vi "Build DashBoard Data.vi"(11 "Dashboard Enables":T3={"Analog Module 1"=[TRUE, TRUE, TRUE, TRUE, TRUE, TRUE, TRUE, TRUE], "Analog Module 2"=[FALSE, FALSE, FALSE, FALSE, FALSE, FALSE, FALSE, FALSE], "Digital Module 1"=TRUE, "Digital Module 2"=FALSE, "Solenoid Module"=TRUE}) -> ()   [LabVIEW 2011]
doc: "This VI builds data and sends it back to the dashboard PC program. By default it sends back the raw values for the first analog, digital, and solenoid module. Modify it to send back the data you want to view. Consider adding higher level data to the Dashboard Datatype.ctl and to this VI. Then update the Dashboard to display the data however you like.\n\nThis software is licensed. Open the labview\\readme\\WPI Robotics Library Open Source License.txt file for more information."
uses:
  DashboardEnable.ctl
  Dashboard Datatype.ctl
  <vilib>/Rock Robotics/WPI/DriverStation/WPI_DriverStationDigitalData.ctl
  <vilib>/Rock Robotics/WPI/DriverStation/DriverStationLCD/WPI_DriverStationLCDLCDLine.ctl
  System Set Points and States.vi
  Robot Global Data.vi
panel:
  out "Dashboard Data":T1
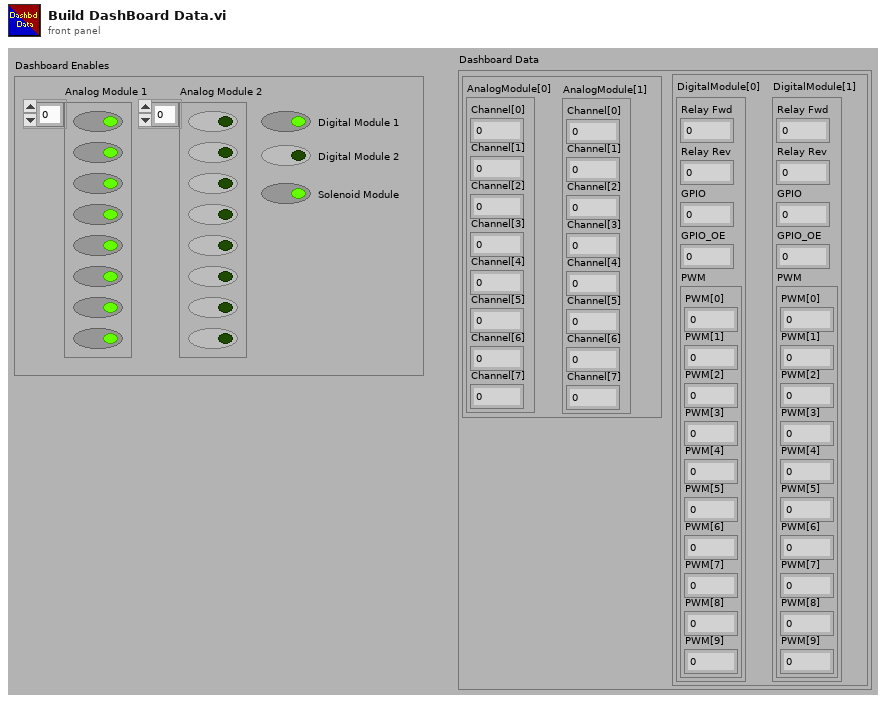
[diagram p1: front panel]
types:
  T1 = typedef "Dashboard Datatype.ctl" = cluster{cluster{"AnalogModule[0]":cluster{"Channel[0]":sgl, "Channel[1]":sgl, "Channel[2]":sgl, "Channel[3]":sgl, "Channel[4]":sgl, "Channel[5]":sgl, "Channel[6]":sgl, "Channel[7]":sgl}, "AnalogModule[1]":cluster{"Channel[0]":sgl, "Channel[1]":sgl, "Channel[2]":sgl, "Channel[3]":sgl, "Channel[4]":sgl, "Channel[5]":sgl, "Channel[6]":sgl, "Channel[7]":sgl}}, cluster{"DigitalModule[0]":T2, "DigitalModule[1]":T2}}
  T2 = typedef "WPI_DriverStationDigitalData.ctl" = cluster{"Relay Fwd":u8, "Relay Rev":u8, "GPIO":u16, "GPIO_OE":u16, "PWM":cluster{"PWM[0]":u8, "PWM[1]":u8, "PWM[2]":u8, "PWM[3]":u8, "PWM[4]":u8, "PWM[5]":u8, "PWM[6]":u8, "PWM[7]":u8, "PWM[8]":u8, "PWM[9]":u8}}
  T3 = typedef "DashboardEnable.ctl" = cluster{"Analog Module 1":bool[], "Analog Module 2":bool[], "Digital Module 1":bool, "Digital Module 2":bool, "Solenoid Module":bool}
  T4 = typedef "WPI_DriverStationLCDLCDLine.ctl" = enum16{"Main - Line 1", "User - Line 2", "User - Line 3", "User - Line 4", "User - Line 5", "User - Line 6"}
  T5 = cluster{"Position":cluster{"X":dbl, "Y":dbl}, "Distance (ft)":dbl}[]
  T6 = cluster{"Target Info[0]":cluster{"Position":cluster{"X":dbl, "Y":dbl}, "Distance (ft)":dbl}, "Target Info[1]":cluster{"Position":cluster{"X":dbl, "Y":dbl}, "Distance (ft)":dbl}, "Target Info[2]":cluster{"Position":cluster{"X":dbl, "Y":dbl}, "Distance (ft)":dbl}, "Target Info[3]":cluster{"Position":cluster{"X":dbl, "Y":dbl}, "Distance (ft)":dbl}, "Target Info[4]":cluster{"Position":cluster{"X":dbl, "Y":dbl}, "Distance (ft)":dbl}, "Target Info[5]":cluster{"Position":cluster{"X":dbl, "Y":dbl}, "Distance (ft)":dbl}, "Target Info[6]":cluster{"Position":cluster{"X":dbl, "Y":dbl}, "Distance (ft)":dbl}, "Target Info[7]":cluster{"Position":cluster{"X":dbl, "Y":dbl}, "Distance (ft)":dbl}, "Target Info[8]":cluster{"Position":cluster{"X":dbl, "Y":dbl}, "Distance (ft)":dbl}}
  T7 = cluster{"AnalogModule[0]":cluster{"Channel[0]":sgl, "Channel[1]":sgl, "Channel[2]":sgl, "Channel[3]":sgl, "Channel[4]":sgl, "Channel[5]":sgl, "Channel[6]":sgl, "Channel[7]":sgl}, "AnalogModule[1]":cluster{"Channel[0]":sgl, "Channel[1]":sgl, "Channel[2]":sgl, "Channel[3]":sgl, "Channel[4]":sgl, "Channel[5]":sgl, "Channel[6]":sgl, "Channel[7]":sgl}}
  T8 = cluster{"Channel[0]":sgl, "Channel[1]":sgl, "Channel[2]":sgl, "Channel[3]":sgl, "Channel[4]":sgl, "Channel[5]":sgl, "Channel[6]":sgl, "Channel[7]":sgl}[]
  T9 = cluster{"Channel[0]":sgl, "Channel[1]":sgl, "Channel[2]":sgl, "Channel[3]":sgl, "Channel[4]":sgl, "Channel[5]":sgl, "Channel[6]":sgl, "Channel[7]":sgl}
  T10 = cluster{"AnalogModule[0][0]":sgl, "AnalogModule[0][1]":sgl, "AnalogModule[0][2]":sgl, "AnalogModule[0][3]":sgl, "AnalogModule[0][4]":sgl, "AnalogModule[0][5]":sgl, "AnalogModule[0][6]":sgl, "AnalogModule[0][7]":sgl}
  T11 = cluster{"[0]":cluster{"Channel[0]":sgl, "Channel[1]":sgl, "Channel[2]":sgl, "Channel[3]":sgl, "Channel[4]":sgl, "Channel[5]":sgl, "Channel[6]":sgl, "Channel[7]":sgl}, "[1]":cluster{"Channel[0]":sgl, "Channel[1]":sgl, "Channel[2]":sgl, "Channel[3]":sgl, "Channel[4]":sgl, "Channel[5]":sgl, "Channel[6]":sgl, "Channel[7]":sgl}}
  T12 = cluster{"DigitalModule[0]":T2, "DigitalModule[1]":T2}
  T13 = typedef "FPGA_DIODevRef.ctl" = cluster{"DevStatus":errorcluster, "Module":T14}
  T14 = typedef "FPGA_TypedefDigitalModule.ctl" = enum16{"Digital Module 1", "Digital Module 2"}
  T15 = cluster{"[0]":u8, "[1]":u8, "[2]":u8, "[3]":u8, "[4]":u8, "[5]":u8, "[6]":u8, "[7]":u8, "[8]":u8, "[9]":u8}
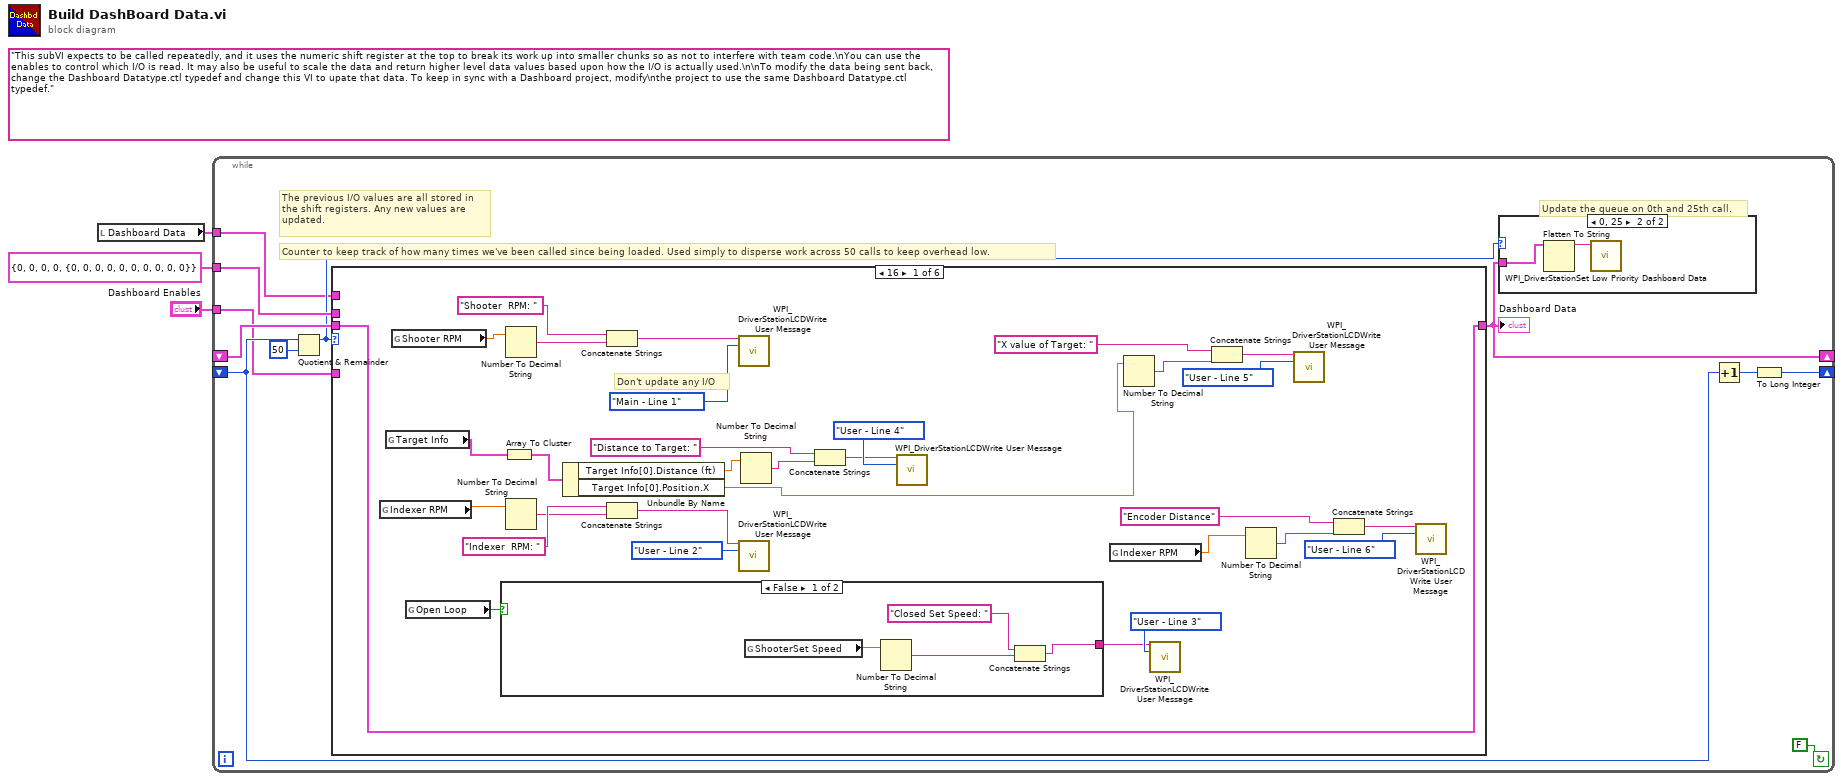
[diagram p0: block diagram]
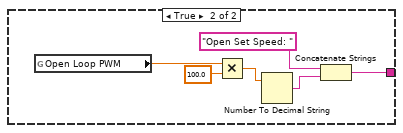
[diagram p3: hidden frame]
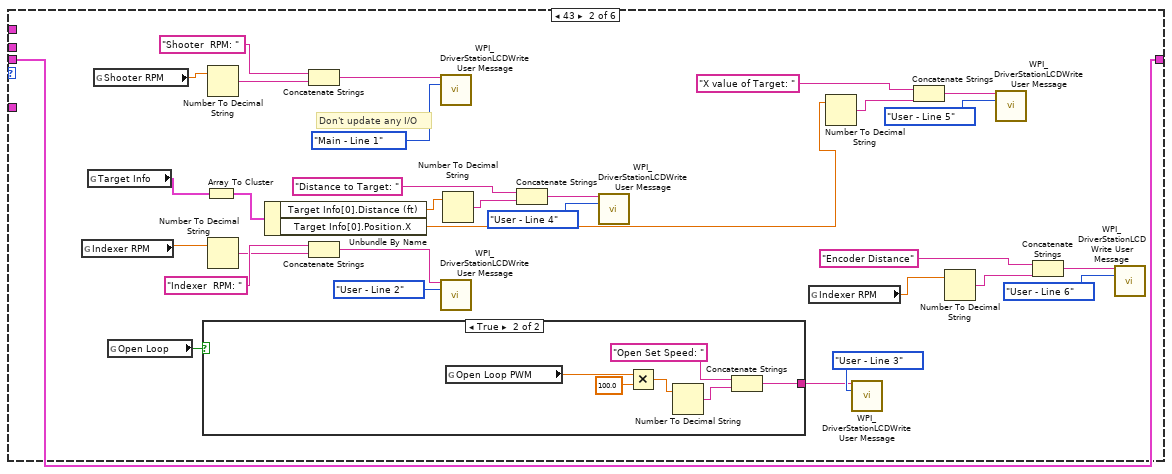
[diagram p4: hidden frame]
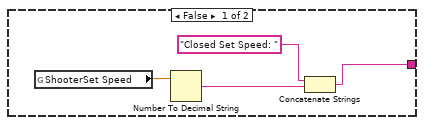
[diagram p5: hidden frame]
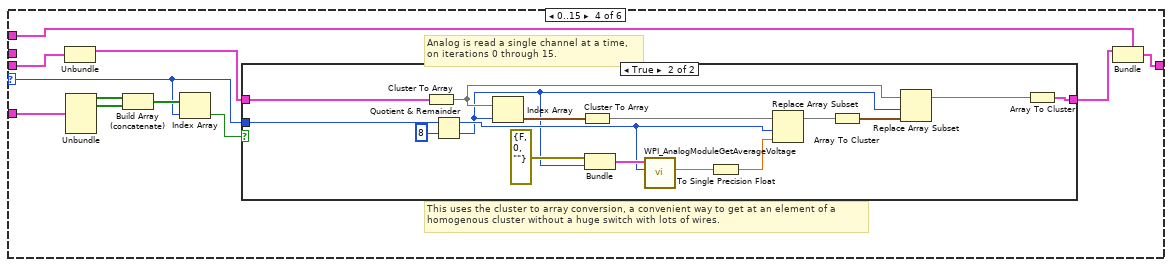
[diagram p7: hidden frame]
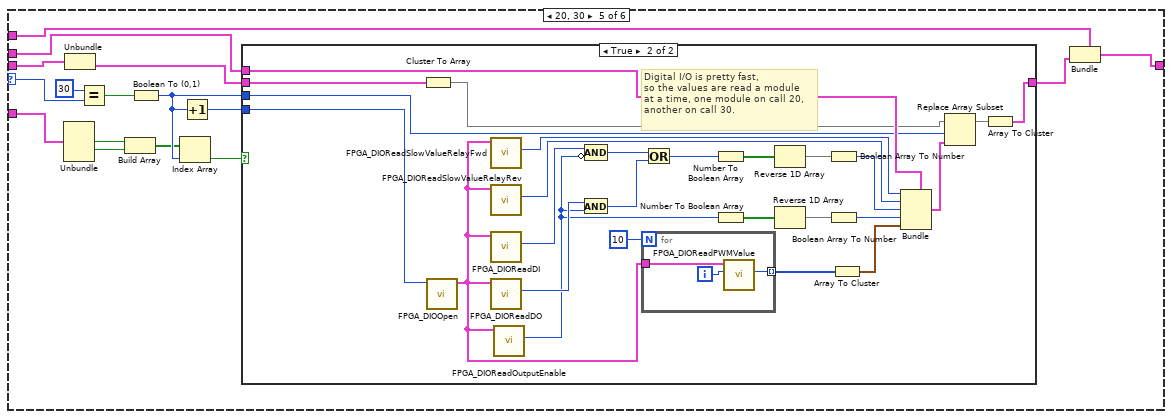
[diagram p9: hidden frame]
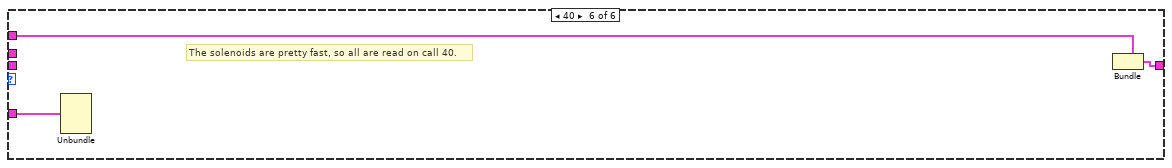
[diagram p11: hidden frame]
diagram:
  (unwired) "This subVI expects to be called repeatedly, and it uses the numeric shift register at the top to break its work up into smaller chunks so as not to interfere with team code.\nYou can use the enables to control which I/O is read. It may also be useful to scale the data and return higher level data values based upon how the I/O is actually used.\n\nTo modify the data being sent back, change the Dashboard Datatype.ctl typedef and change this VI to upate that data. To keep in sync with a Dashboard project, modify\nthe project to use the same Dashboard Datatype.ctl typedef."
  n1 = local read "Dashboard Data"() -> (w2:T1)
  n2 = while {
    shift-right: [w7] -> _
    shift-left: _ -> [w9]
    shift-right: [w4] -> _
    shift-left: _ -> [w12]
    tunnel: T2 {"Relay Fwd"=0, "Relay Rev"=0, "GPIO"=0, "GPIO_OE"=0, "PWM"={"PWM[0]"=0, "PWM[1]"=0, "PWM[2]"=0, "PWM[3]"=0, "PWM[4]"=0, "PWM[5]"=0, "PWM[6]"=0, "PWM[7]"=0, "PWM[8]"=0, "PWM[9]"=0}} ("DigitalModule[1]") -> [w11]
    tunnel: w2 -> [w6]
    tunnel: "Dashboard Enables" -> [w5]
    stop <- FALSE continue-if-true
    # "Counter to keep track of how many times we've been called since being loaded. Used simply to disperse work across 50 calls to keep overhead low."
    # "Update the queue on 0th and 25th call."
    # "The previous I/O values are all stored in\nthe shift registers. Any new values are\nupdated."
    n3 = Quotient & Remainder(x=w9, y=50) -> (x-y*floor(x/y)=w8:i32)  [unwired: 1 out]
    n4 = case shown="16" w8 {
      selector: w8 -> [_ _ _ w105 w137 _]
      tunnel: [w47 w63 w99 w101 w128 w175] -> w4
      tunnel: w12 -> [w47 w63 w99 w100 w130 _]
      tunnel: w11 -> [_ _ _ _ w143 _]
      tunnel: w6 -> [_ _ _ w107 w129 w174]
      tunnel: w5 -> [_ _ _ w104 w135 w176]
      frame 16 {
        # "Don't update any I/O"
        n5 = global read "System Set Points and States.vi" "Indexer RPM"() -> (w31:dbl)
        n6 = global read "Robot Global Data.vi" "Target Info"() -> (w39:T5)
        n7 = global read "System Set Points and States.vi" "Shooter RPM"() -> (w30:dbl)
        n8 = global read "System Set Points and States.vi" "Open Loop"() -> (w46:bool)
        n9 = case shown="False" w46 {
          tunnel: [w50 w57] -> w44
          frame False {
            n10 = global read "System Set Points and States.vi" "ShooterSet Speed"() -> (w48:dbl)
            n11 = Number To Decimal String(number=w48) -> (decimal integer string=w49:string)  [unwired: 1 in]
            n12 = Concatenate Strings("Closed Set Speed: ", w49) -> (w50:string)
          }
          frame True {
            n13 = global read "System Set Points and States.vi" "Open Loop PWM"() -> (w56:dbl)
            n14 = Multiply(x=w56, y=100.0) -> (x*y=w52:dbl)
            n15 = Number To Decimal String(number=w52) -> (decimal integer string=w53:string)  [unwired: 1 in]
            n16 = Concatenate Strings("Open Set Speed: " ("string"), w53) -> (w57:string)
          }
        }
        n17 = Array To Cluster(array=w39) -> (cluster=w26:T6)
        n18 = Number To Decimal String(number=w30) -> (decimal integer string=w40:string)  [unwired: 1 in]
        n19 = Number To Decimal String(number=w31) -> (decimal integer string=w32:string)  [unwired: 1 in]
        n20 = Unbundle By Name(w26) -> ("Target Info[0].Distance (ft)"=w23:dbl, "Target Info[0].Position.X"=w25:dbl)
        n21 = Concatenate Strings("Shooter  RPM: ", w40) -> (w42:string)
        n22 = Concatenate Strings("Indexer  RPM: ", w32) -> (w34:string)
        n23 = call <vilib>:"WPI_DriverStationLCDWrite User Message.vi"("line text"=w42, "line"=WPI_DriverStationLCDLCDLine."Main - Line 1") -> ()  [unwired: 13 in, 1 out]
        n24 = call <vilib>:"WPI_DriverStationLCDWrite User Message.vi"("line text"=w34, "line"=WPI_DriverStationLCDLCDLine."User - Line 2") -> ()  [unwired: 13 in, 1 out]
        n25 = Number To Decimal String(number=w23) -> (decimal integer string=w22:string)  [unwired: 1 in]
        n26 = Concatenate Strings("Distance to Target: " ("string"), w22) -> (w36:string)
        n27 = call <vilib>:"WPI_DriverStationLCDWrite User Message.vi"("line text"=w36, "line"=WPI_DriverStationLCDLCDLine."User - Line 4") -> ()  [unwired: 13 in, 1 out]
        n28 = global read "System Set Points and States.vi" "Indexer RPM"() -> (w17:dbl)
        n29 = Number To Decimal String(number=w25) -> (decimal integer string=w24:string)  [unwired: 1 in]
        n30 = call <vilib>:"WPI_DriverStationLCDWrite User Message.vi"("line text"=w44, "line"=WPI_DriverStationLCDLCDLine."User - Line 3") -> ()  [unwired: 13 in, 1 out]
        n31 = Concatenate Strings("X value of Target: " ("string"), w24) -> (w27:string)
        n32 = Number To Decimal String(number=w17) -> (decimal integer string=w18:string)  [unwired: 1 in]
        n33 = call <vilib>:"WPI_DriverStationLCDWrite User Message.vi"("line text"=w27, "line"=WPI_DriverStationLCDLCDLine."User - Line 5") -> ()  [unwired: 13 in, 1 out]
        n34 = Concatenate Strings("Encoder Distance" ("string"), w18) -> (w19:string)
        n35 = call <vilib>:"WPI_DriverStationLCDWrite User Message.vi"("line text"=w19, "line"=WPI_DriverStationLCDLCDLine."User - Line 6") -> ()  [unwired: 13 in, 1 out]
      }
      frame 43 {
        # "Don't update any I/O"
        n36 = global read "System Set Points and States.vi" "Indexer RPM"() -> (w73:dbl)
        n37 = global read "Robot Global Data.vi" "Target Info"() -> (w81:T5)
        n38 = global read "System Set Points and States.vi" "Shooter RPM"() -> (w72:dbl)
        n39 = global read "System Set Points and States.vi" "Open Loop"() -> (w88:bool)
        n40 = case shown="True" w88 {
          tunnel: [w89 w98] -> w86
          frame False {
            n41 = global read "System Set Points and States.vi" "ShooterSet Speed"() -> (w90:dbl)
            n42 = Number To Decimal String(number=w90) -> (decimal integer string=w91:string)  [unwired: 1 in]
            n43 = Concatenate Strings("Closed Set Speed: ", w91) -> (w89:string)
          }
          frame True {
            n44 = global read "System Set Points and States.vi" "Open Loop PWM"() -> (w97:dbl)
            n45 = Multiply(x=w97, y=100.0) -> (x*y=w93:dbl)
            n46 = Number To Decimal String(number=w93) -> (decimal integer string=w94:string)  [unwired: 1 in]
            n47 = Concatenate Strings("Open Set Speed: " ("string"), w94) -> (w98:string)
          }
        }
        n48 = Array To Cluster(array=w81) -> (cluster=w68:T6)
        n49 = Number To Decimal String(number=w72) -> (decimal integer string=w82:string)  [unwired: 1 in]
        n50 = Number To Decimal String(number=w73) -> (decimal integer string=w74:string)  [unwired: 1 in]
        n51 = Unbundle By Name(w68) -> ("Target Info[0].Distance (ft)"=w65:dbl, "Target Info[0].Position.X"=w67:dbl)
        n52 = Concatenate Strings("Shooter  RPM: ", w82) -> (w84:string)
        n53 = Concatenate Strings("Indexer  RPM: ", w74) -> (w76:string)
        n54 = call <vilib>:"WPI_DriverStationLCDWrite User Message.vi"("line text"=w84, "line"=WPI_DriverStationLCDLCDLine."Main - Line 1") -> ()  [unwired: 13 in, 1 out]
        n55 = call <vilib>:"WPI_DriverStationLCDWrite User Message.vi"("line text"=w76, "line"=WPI_DriverStationLCDLCDLine."User - Line 2") -> ()  [unwired: 13 in, 1 out]
        n56 = Number To Decimal String(number=w65) -> (decimal integer string=w64:string)  [unwired: 1 in]
        n57 = Concatenate Strings("Distance to Target: " ("string"), w64) -> (w78:string)
        n58 = call <vilib>:"WPI_DriverStationLCDWrite User Message.vi"("line text"=w78, "line"=WPI_DriverStationLCDLCDLine."User - Line 4") -> ()  [unwired: 13 in, 1 out]
        n59 = global read "System Set Points and States.vi" "Indexer RPM"() -> (w58:dbl)
        n60 = Number To Decimal String(number=w67) -> (decimal integer string=w66:string)  [unwired: 1 in]
        n61 = call <vilib>:"WPI_DriverStationLCDWrite User Message.vi"("line text"=w86, "line"=WPI_DriverStationLCDLCDLine."User - Line 3") -> ()  [unwired: 13 in, 1 out]
        n62 = Concatenate Strings("X value of Target: " ("string"), w66) -> (w69:string)
        n63 = Number To Decimal String(number=w58) -> (decimal integer string=w59:string)  [unwired: 1 in]
        n64 = call <vilib>:"WPI_DriverStationLCDWrite User Message.vi"("line text"=w69, "line"=WPI_DriverStationLCDLCDLine."User - Line 5") -> ()  [unwired: 13 in, 1 out]
        n65 = Concatenate Strings("Encoder Distance" ("string"), w59) -> (w60:string)
        n66 = call <vilib>:"WPI_DriverStationLCDWrite User Message.vi"("line text"=w60, "line"=WPI_DriverStationLCDLCDLine."User - Line 6") -> ()  [unwired: 13 in, 1 out]
      }
      frame Default {
      }
      frame 0..15 {
        # "This uses the cluster to array conversion, a convenient way to get at an element of a\nhomogenous cluster without a huge switch with lots of wires."
        # "Analog is read a single channel at a time,\non iterations 0 through 15."
        n67 = Unbundle(w100) -> (w106:T7)  [unwired: 1 out]
        n68 = Unbundle(w104) -> ("Analog Module 1"=w103:bool[], "Analog Module 2"=w102:bool[])  [unwired: 3 out]
        n69 = Build Array (concatenate)(w103, w102) -> (w109:bool[])
        n70 = Index Array(array=w109, index=w105) -> (element=w110:bool)
        n71 = case shown="True" w110 {
          tunnel: w105 -> [_ w118]
          tunnel: [w111 w115] -> w108
          tunnel: w106 -> [w111 w114]
          frame False {
          }
          frame True {
            n72 = Cluster To Array(cluster=w114) -> (array=w113:T8)
            n73 = Quotient & Remainder(x=w118, y=8) -> (x-y*floor(x/y)=w117:i32, floor(x/y)=w112:i32)
            n74 = Index Array(array=w113, index=w112) -> (element=w120:T9)
            n75 = Cluster To Array(cluster=w120) -> (array=w119:sgl[])
            n76 = Bundle("DevStatus"=errorcluster {"status"=FALSE, "code"=0, "source"=""}, w112) -> (w126:cluster{"DevStatus":errorcluster, i32})  [unwired: 1 out]
            n77 = call <vilib>:"WPI_AnalogModuleGetAverageVoltage.vi"("Channel"=w117, "AnalogModuleDevStatus"=w126) -> ("Average Voltage"=w123:dbl)  [unwired: 1 in, 8 out]
            n78 = To Single Precision Float(number=w123) -> (single precision float=w122:sgl)
            n79 = Replace Array Subset(array=w119, new element=w122, index=w117) -> (w121:sgl[])
            n80 = Array To Cluster(array=w121) -> (cluster=w125:T10)
            n81 = Replace Array Subset(array=w113, new element=w125, index=w112) -> (w116:T8)
            n82 = Array To Cluster(array=w116) -> (cluster=w115:T11)
          }
        }
        n83 = Bundle(cluster=w107, w108) -> (w101:T1)  [unwired: 1 out]
      }
      frame 20, 30 {
        n84 = Unbundle(w135) -> ("Digital Module 1"=w134:bool, "Digital Module 2"=w133:bool)  [unwired: 3 out]
        n85 = Unbundle(w130) -> (w132:T12)  [unwired: 1 out]
        n86 = Equal?(x=30, y=w137) -> (x = y?=w141:bool)
        n87 = Build Array(w134, w133) -> (w136:bool[])
        n88 = Boolean To (0,1)(Boolean=w141) -> (0, 1=w139:i16)
        n89 = Index Array(array=w136, index=w139) -> (element=w138:bool)
        n90 = Increment(x=w139) -> (x+1=w140:i16)
        n91 = case shown="True" w138 {
          tunnel: w143 -> [_ w152]
          tunnel: [w144 w145] -> w131
          tunnel: w140 -> [_ w150]
          tunnel: w139 -> [_ w149]
          tunnel: w132 -> [w144 w148]
          frame False {
          }
          frame True {
            # "Digital I/O is pretty fast,\nso the values are read a module\nat a time, one module on call 20,\nanother on call 30."
            n92 = Cluster To Array(cluster=w148) -> (array=w147:T2[])
            n93 = call <vilib>:"FPGA_DIOOpen.vi"("Module (Module 1)"=w150) -> ("DIODeviceRef"=w168:T13)  [unwired: 1 in, 9 out]
            n94 = call <vilib>:"FPGA_DIOReadSlowValueRelayFwd.vi"("DIODeviceRef In"=w168) -> ("Relay Forward"=w161:u8)  [unwired: 1 in, 9 out]
            n95 = call <vilib>:"FPGA_DIOReadSlowValueRelayRev.vi"("DIODeviceRef In"=w168) -> ("Relay Reverse"=w162:u8)  [unwired: 1 in, 9 out]
            n96 = call <vilib>:"FPGA_DIOReadDI.vi"("DIODeviceRef In"=w168) -> ("DI"=w166:u16)  [unwired: 1 in, 9 out]
            n97 = call <vilib>:"FPGA_DIOReadDO.vi"("DIODeviceRef In"=w168) -> ("DO"=w165:u16)  [unwired: 1 in, 9 out]
            n98 = call <vilib>:"FPGA_DIOReadOutputEnable.vi"("DIODeviceRef In"=w168) -> ("OutputEnable"=w156:u16)  [unwired: 1 in, 9 out]
            n99 = And(x=w165, y=w156) -> (x .and. y?=w164:u16)
            n100 = Compound Arithmetic op=AND(w166, invert w156) -> (w163:u16)
            n101 = for {
              N: 10 -> [_]
              tunnel: w168 -> [w173]
              tunnel: [w171] -> w169 mode=indexing
              i -> [w172]
              n102 = call <vilib>:"FPGA_DIOReadPWMValue.vi"("PWMChannel"=w172, "DIODeviceRef In"=w173) -> ("PWMValue"=w171:u8)  [unwired: 1 in, 8 out]
            }
            n103 = Or(x=w163, y=w164) -> (x .or. y?=w154:u16)
            n104 = Number To Boolean Array(number=w154) -> (Boolean array=w159:bool[])
            n105 = Number To Boolean Array(number=w156) -> (Boolean array=w158:bool[])
            n106 = Reverse 1D Array(array=w159) -> (reversed array=w160:bool[])
            n107 = Reverse 1D Array(array=w158) -> (reversed array=w157:bool[])
            n108 = Boolean Array To Number(Boolean array=w160) -> (number=w153:u32)
            n109 = Boolean Array To Number(Boolean array=w157) -> (number=w155:u32)
            n110 = Array To Cluster(array=w169) -> (cluster=w167:T15)
            n111 = Bundle(cluster=w152, "Relay Fwd"=w161, "Relay Rev"=w162, "GPIO"=w153, "GPIO_OE"=w155, "PWM"=w167) -> (w151:T2)
            n112 = Replace Array Subset(array=w147, new element=w151, index=w149) -> (w146:T2[])
            n113 = Array To Cluster(array=w146) -> (cluster=w145:cluster{"[0]":T2, "[1]":T2})
          }
        }
        n114 = Bundle(cluster=w129, w131) -> (w128:T1)  [unwired: 1 out]
      }
      frame 40 {
        # "The solenoids are pretty fast, so all are read on call 40."
        n115 = Unbundle(w176) -> ()  [unwired: 5 out]
        n116 = Bundle(cluster=w174) -> (w175:T1)  [unwired: 2 out]
      }
    }
    "Dashboard Data" <- w4
    n117 = case shown="0, 25" w8 {
      tunnel: w4 -> [_ w16]
      frame Default {
      }
      frame 0, 25 {
        n118 = Flatten To String(anything=w16) -> (data string=w15:string)  [unwired: 1 in, 4 out]
        n119 = call <vilib>:"WPI_DriverStationSet Low Priority Dashboard Data.vi"("User Data"=w15) -> ()  [unwired: 1 in, 10 out]
      }
    }
    n120 = Increment(x=w9) -> (x+1=w14:i32)
    n121 = To Long Integer(number=w14) -> (32bit integer=w7:i32)
  }
